vi "dActivationFunction.vi"(11 "Output":sgl) -> (3 "f":sgl)   [LabVIEW 2020]
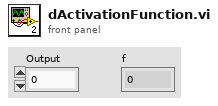
[diagram p1: front panel]
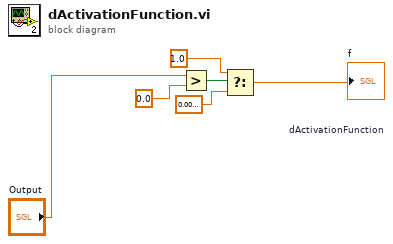
[diagram p0: block diagram]
diagram:
  n1 = Greater?(x="Output", y=sgl 0.0 ("f")) -> (0:w4:bool)
  n2 = Select "dActivationFunction"(t=sgl 1.0, s=w4, f=sgl 0.01) -> (s? t:f=→"f":sgl)
